vi "GET BLISS Filter Dates.vi"(7 "Data Parameters in":T1={"Forces in Theater"=[{"Force Commander"="BlissUT124", "Units"=[]}, {"Force Commander"="BlissMP146", "Units"=[]}, {"Force Commander"="BlissMP145", "Units"=[]}, {"Force Commander"="BlissMP140", "Units"=[]}, {"Force Commander"="BlissMP137", "Units"=[]}, {"Force Commander"="BlissMP135", "Units"=[]}, {"Force Commander"="BlissMP134", "Units"=[]}, {"Force Commander"="BlissMP132", "Units"=[]}, {"Force Commander"="BlissMA109", "Units"=[]}, {"Force Commander"="BlissMA107", "Units"=[]}, {"Force Commander"="BlissMA106", "Units"=[]}, {"Force Commander"="BlissMA101", "Units"=[]}, {"Force Commander"="BlissLU118", "Units"=[]}, {"Force Commander"="BlissLU117", "Units"=[]}, {"Force Commander"="BlissLU116", "Units"=[]}, {"Force Commander"="BlissLU115", "Units"=[]}, {"Force Commander"="BlissLU114", "Units"=[]}, {"Force Commander"="BlissLU113", "Units"=[]}, {"Force Commander"="BlissLU111", "Units"=[]}, {"Force Commander"="BlissLL185", "Units"=[]}, {"Force Commander"="BlissLL183", "Units"=[]}, {"Force Commander"="BlissLL173", "Units"=[]}, {"Force Commander"="BlissLL172", "Units"=[]}, {"Force Commander"="BlissLL171", "Units"=[]}, {"Force Commander"="BlissJH103", "Units"=[]}, {"Force Commander"="BlissJH102", "Units"=[]}, {"Force Commander"="BlissJH101", "Units"=[]}, {"Force Commander"="BlissJE116", "Units"=[]}, {"Force Commander"="BlissJE115", "Units"=[]}, {"Force Commander"="BlissJE114", "Units"=[]}, {"Force Commander"="BlissJE111", "Units"=[]}, {"Force Commander"="BlissHD183", "Units"=[]}, {"Force Commander"="BlissHD182", "Units"=[]}, {"Force Commander"="BlissHD181", "Units"=[]}, {"Force Commander"="BlissGPDFFPL", "Units"=[]}, {"Force Commander"="BlissEUWIPES", "Units"=[]}, {"Force Commander"="BlissEU179", "Units"=[]}, {"Force Commander"="BlissEU178", "Units"=[]}, {"Force Commander"="BlissEU177", "Units"=[]}, {"Force Commander"="Blissdvds02", "Units"=[]}, {"Force Commander"="BlissDOWIPES", "Units"=[]}, {"Force Commander"="BlissCR022", "Units"=[]}, {"Force Commander"="BlissCR021", "Units"=[]}, {"Force Commander"="BlissCG167", "Units"=[]}, {"Force Commander"="BlissCG166", "Units"=[]}, {"Force Commander"="BlissCG161", "Units"=[]}, {"Force Commander"="BlissCG160", "Units"=[]}, {"Force Commander"="BlissCG159", "Units"=[]}, {"Force Commander"="BlissCG158", "Units"=[]}, {"Force Commander"="BlissCG157", "Units"=[]}, {"Force Commander"="BlissCG156", "Units"=[]}, {"Force Commander"="BlissCG151", "Units"=[]}, {"Force Commander"="BlissCB172", "Units"=[]}, {"Force Commander"="BlissCB171", "Units"=[]}, {"Force Commander"="BlissCB108", "Units"=[]}, {"Force Commander"="BlissCB107", "Units"=[]}, {"Force Commander"="BlissBV181", "Units"=[]}, {"Force Commander"="BlissBV162", "Units"=[]}, {"Force Commander"="BlissAK177", "Units"=[]}, {"Force Commander"="BlissAK176", "Units"=[]}, {"Force Commander"="BlissAK175", "Units"=[]}, {"Force Commander"="BlissAK174", "Units"=[]}, {"Force Commander"="BlissAK173", "Units"=[]}, {"Force Commander"="BlissAK172", "Units"=[]}, {"Force Commander"="BlissAK171", "Units"=[]}, {"Force Commander"="BlissAK139", "Units"=[]}, {"Force Commander"="BlissAK134", "Units"=[]}, {"Force Commander"="BlissAK131", "Units"=[]}, {"Force Commander"="BlissAH163", "Units"=[]}, {"Force Commander"="BlissAH162", "Units"=[]}, {"Force Commander"="BlissAH161", "Units"=[]}, {"Force Commander"="BlissAH122", "Units"=[]}, {"Force Commander"="BlissAH121", "Units"=[]}, {"Force Commander"="BlissAD106", "Units"=[]}, {"Force Commander"="BlissAD104", "Units"=[]}, {"Force Commander"="BlissAB105", "Units"=[]}, {"Force Commander"="BlissAB104", "Units"=[]}]}, 8 "error in":errorcluster, 9 "Dates (folders)":string[](array[string]), 11 "Server Images Path":path) -> (0 "error out":errorcluster, 1 "Valid Dates":string[](array[string]), 3 "Valid Paths":path[](array[path]))   [LabVIEW 2020]
uses:
  MC5e Squad_Info.ctl
  MC5e Squad_Set.ctl
  MC5e Data_Parameters.ctl
  MC5e Terrain types.ctl
  Location.ctl
  MC5e Unit.ctl
  MC5e Force.ctl
  MC5e Size_Categories.ctl
panel:
  # "Squads are restricted to one type of soldier (i.e  Archers) and all of the same level.\nIf you want mixed CR or mixed types, use multiple squads."
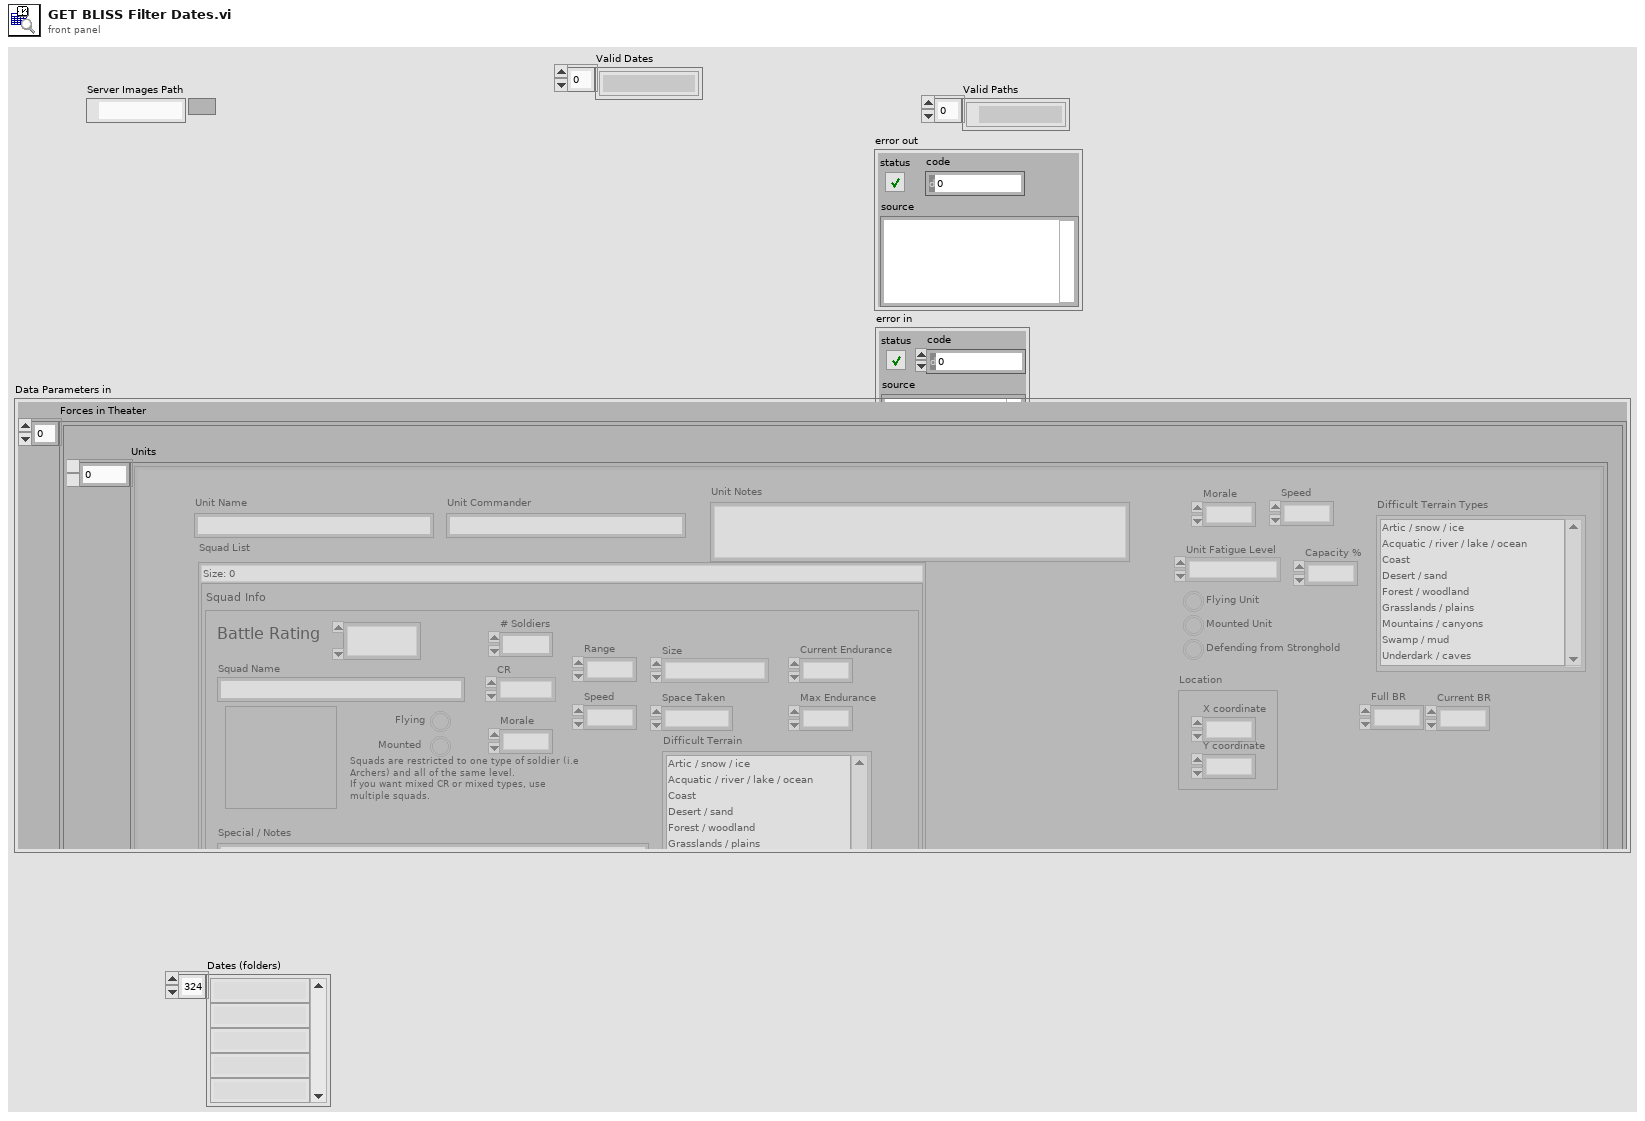
[diagram p1: front panel]
types:
  T1 = typedef "MC5e Data_Parameters.ctl" = cluster{"Forces in Theater":T2[]}
  T2 = typedef "MC5e Force.ctl" = cluster{"Force Commander":string, "Units":T3[]}
  T3 = typedef "MC5e Unit.ctl" = cluster{"Squad List":T4, "Unit Fatigue Level":enum16{"Not Fatigued", "Fatigued", "Seriously Fatigued"}, "Flying Unit":bool, "Mounted Unit":bool, "Difficult Terrain Types":T7, "Full BR":dbl, "Defending from Stronghold":bool, "Speed":dbl, "Capacity %":dbl, "Morale":dbl, "Current BR":dbl, "Location":T8, "Unit Name":string, "Unit Commander":string, "Unit Notes":string}
  T4 = typedef "MC5e Squad_Set.ctl" = set{T5}
  T5 = typedef "MC5e Squad_Info.ctl" = cluster{"Squad Name":string, "# Soldiers":u16, "Battle Rating":u16, "Flying":bool, "Mounted":bool, "Speed":u16, "Range":u16, "Morale":i32, "Token Image":variant, "Max Endurance":u16, "Current Endurance":i32, "Size":T6, "Space Taken":u16, "Difficult Terrain":i32[], "CR":u16, "Special / Notes":string}
  T6 = typedef "MC5e Size_Categories.ctl" = enum16{"Tiny", "Small", "Medium", "Large", "Huge", "Gargantuan"}
  T7 = typedef "MC5e Terrain types.ctl" = i32[]
  T8 = typedef "Location.ctl" = cluster{"X coordinate":dbl, "Y coordinate":dbl}
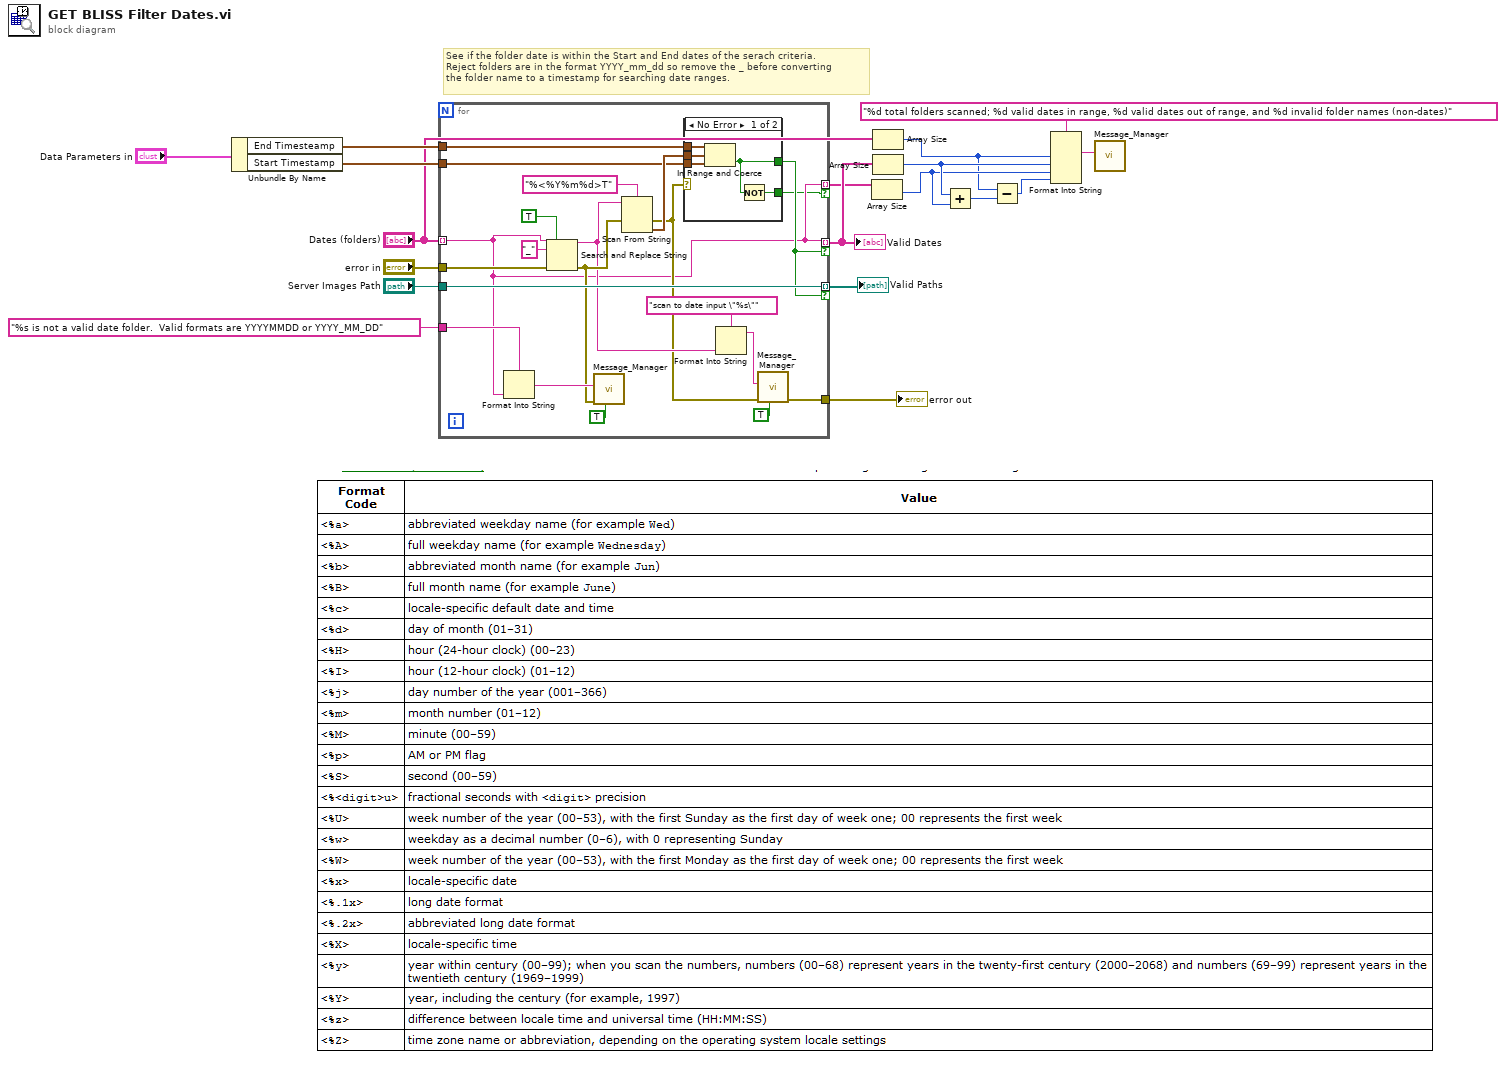
[diagram p0: block diagram]
diagram:
  # "See if the folder date is within the Start and End dates of the serach criteria.\nReject folders are in the format YYYY_mm_dd so remove the _ before converting\nthe folder name to a timestamp for searching date ranges."
  n1 = Unbundle By Name("Data Parameters in") -> ("End Timesteamp"=w16:timestamp, "Start Timestamp"=w15:timestamp)
  n2 = for {
    tunnel: "Dates (folders)" -> [w20] mode=indexing
    tunnel: [w20] -> w11 mode=indexing if=w31
    tunnel: "error in" -> [w39]
    tunnel: "Server Images Path" -> [w32]
    tunnel: w16 -> [w34]
    tunnel: w15 -> [w33]
    tunnel: [w32] -> w14 mode=indexing if=w31
    tunnel: "%s is not a valid date folder.  Valid formats are YYYYMMDD or YYYY_MM_DD" ("format string") -> [w28]
    tunnel: [w21] -> w8
    tunnel: [w20] -> w7 mode=indexing if=w19
    n3 = Format Into String(format string=w28, w20) -> (resulting string=w30:string)  [unwired: 2 in, 1 out]
    n4 = Search and Replace String(replace all?=TRUE ("replace all? (F)"), input string=w20, search string="_", error in=w39) -> (result string=w25:string, error out=w27:errorcluster)  [unwired: 4 in, 2 out]
    n5 = call "Message_Manager.vi"("Log only on Err"=TRUE ("Log Even if No Error (T)"), "error in"=w27, "New Entry"=w30) -> ()  [unwired: 4 in, 5 out]
    n6 = Scan From String(format string="%<%Y%m%d>T", input string=w25, error in=w27) -> (error out=w22:errorcluster, output 1=w35:timestamp)  [unwired: 2 in, 2 out]
    n7 = case shown="No Error" w22 {
      tunnel: w35 -> [w44 _]
      tunnel: w34 -> [w43 _]
      tunnel: w33 -> [w42 _]
      tunnel: [w41 _] -> w31
      tunnel: [w40 _] -> w19
      frame No Error {
        n8 = In Range and Coerce(upper limit=w43, x=w44, lower limit=w42) -> (In Range?=w41:bool)  [unwired: 1 out]
        n9 = Not(x=w41) -> (.not. x?=w40:bool)
      }
      frame Error {
      }
    }
    n10 = Format Into String(format string="scan to date input \"%s\"", w25) -> (resulting string=w23:string)  [unwired: 2 in, 1 out]
    n11 = call "Message_Manager.vi"("Log only on Err"=TRUE ("Log Even if No Error (T)"), "error in"=w22, "New Entry"=w23) -> ("error out"=w21:errorcluster)  [unwired: 4 in, 4 out]
  }
  "Valid Paths" <- w14
  "Valid Dates" <- w11
  "error out" <- w8
  n12 = Array Size(array=w7) -> (size(s)=w4:i32)
  n13 = Array Size(array="Dates (folders)") -> (size(s)=w2:i32)
  n14 = Array Size(array=w11) -> (size(s)=w5:i32)
  n15 = Add(x=w5, y=w4) -> (x+y=w3:i32)
  n16 = Subtract(x=w2, y=w3) -> (x-y=w1:i32)
  n17 = Format Into String(format string="%d total folders scanned; %d valid dates in range, %d valid dates out of range, and %d invalid folder names (non-dates)", w2, w5, w4, w1) -> (resulting string=w10:string)  [unwired: 2 in, 1 out]
  n18 = call "Message_Manager.vi"("New Entry"=w10) -> ()  [unwired: 6 in, 5 out]
